vi "Detect (SubVI).vi"(9 "Фильтр":bool, 10 "Array in":dbl[](array[numeric]), 11 "length":i32) -> (3 "Array out":dbl[](array[numeric]))   [LabVIEW 2017]
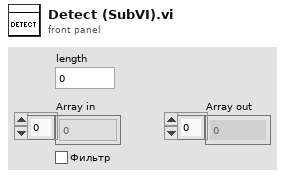
[diagram p1: front panel]
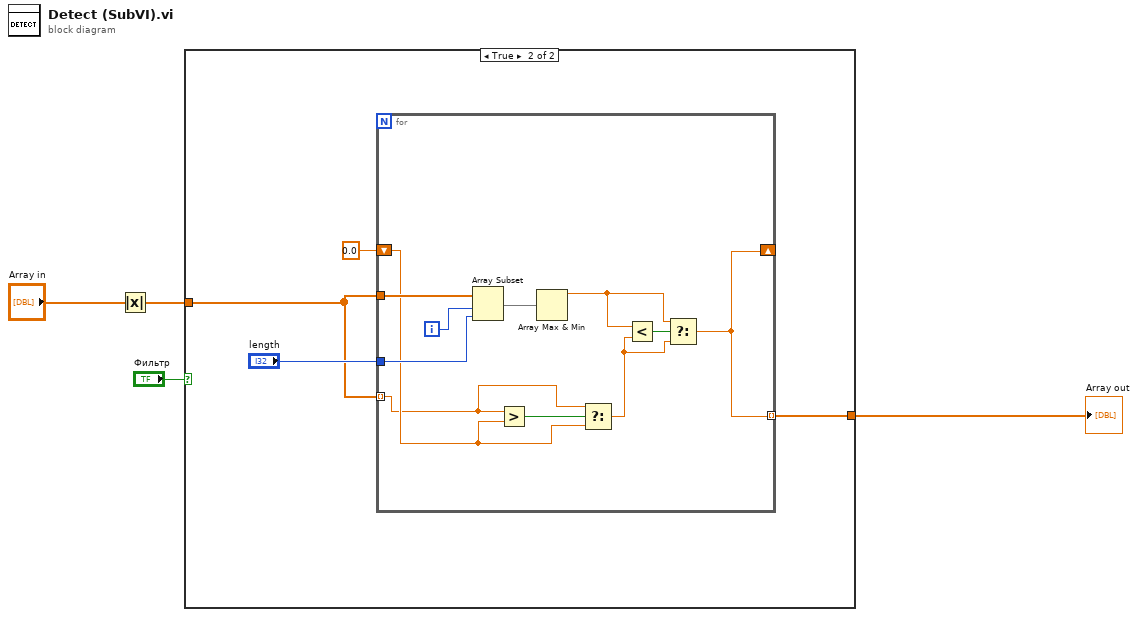
[diagram p0: block diagram]
diagram:
  n1 = Absolute Value(x="Array in") -> (abs(x)=w4:dbl[])
  n2 = case shown="True" "Фильтр" {
    tunnel: w4 -> [w5 w8]
    tunnel: [w5 w7] -> w1
    frame False {
    }
    frame True {
      n3 = for {
        tunnel: w8 -> [w10] mode=indexing
        shift-right: [w16] -> _
        shift-left: 0.0 -> [w11]
        tunnel: [w16] -> w7 mode=indexing
        tunnel: w8 -> [w13]
        tunnel: "length" -> [w12]
        i -> [w19]
        n4 = Array Subset(array=w13, index=w19, length=w12) -> (w18:dbl[])
        n5 = Greater?(x=w10, y=w11) -> (0:w20:bool)
        n6 = Array Max & Min(array=w18) -> (max value=w14:dbl)  [unwired: 3 out]
        n7 = Select(t=w10, s=w20, f=w11) -> (s? t:f=w17:dbl)
        n8 = Less?(x=w14, y=w17) -> (x < y?=w15:bool)
        n9 = Select(t=w14, s=w15, f=w17) -> (s? t:f=w16:dbl)
      }
    }
  }
  "Array out" <- w1
